vi "debug.vi"() -> ()   [LabVIEW 2010, in "LASA Beta.lvrbt"]
uses:
  LASA Beta.lvrbt
  <vilib>/NXT/Block Support/NXT_ButtonSelector.ctl
  <vilib>/NXT/Dual Mode Library/Display/clearDisplay.vi
  <vilib>/NXT/Dual Mode Library/Display/drawText.vi
  <vilib>/NXT/Dual Mode Library/Sensors/readNXTButton.vi
  op-run.vi
  <vilib>/NXT/Dual Mode Library/prims/inRangeAndCoerce/inRangeAndCoerce_float.vi
panel:
  in  "Manipulator position":dbl=127.0
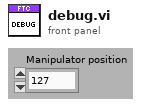
[diagram p1: front panel]
types:
  T1 = typedef "LVHSConnector.ctl" = cluster{"Hardware":string, "Flattened String":string}
  T2 = typedef "NXT_ButtonSelector.ctl" = u16
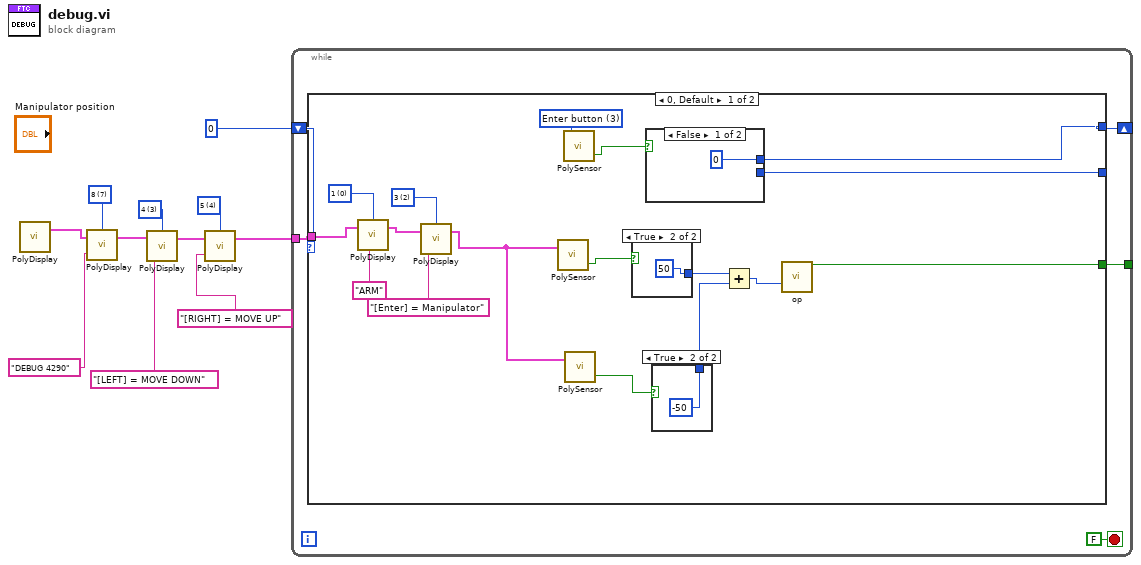
[diagram p0: block diagram]
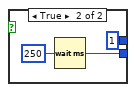
[diagram p4: hidden frame]
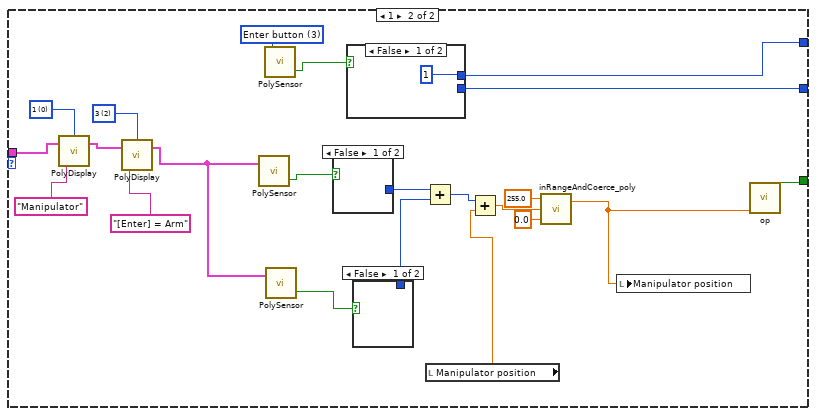
[diagram p5: hidden frame]
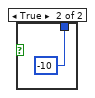
[diagram p6: hidden frame]
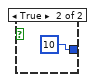
[diagram p7: hidden frame]
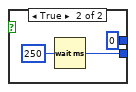
[diagram p8: hidden frame]
diagram:
  w6 = i16 7 items=["1", "2", "3", "4", "5", "6", "7", "8"] ("Line")
  w7 = i16 3 items=["1", "2", "3", "4", "5", "6", "7", "8"] ("Line")
  w8 = i16 4 items=["1", "2", "3", "4", "5", "6", "7", "8"] ("Line")
  n1 = call-poly <vilib>:"PolyDisplay.vi"() -> ("NXT"=w11:T1)  [unwired: 4 in]
  n2 = call-poly <vilib>:"PolyDisplay.vi"("Text"="DEBUG 4290", "NXT"=w11, "Line"=w6) -> ("NXT"=w10:T1)  [unwired: 1 in]
  n3 = call-poly <vilib>:"PolyDisplay.vi"("Text"="[LEFT] = MOVE DOWN", "NXT"=w10, "Line"=w7) -> ("NXT"=w9:T1)  [unwired: 1 in]
  n4 = call-poly <vilib>:"PolyDisplay.vi"("Text"="[RIGHT] = MOVE UP", "NXT"=w9, "Line"=w8) -> ("NXT"=w1:T1)  [unwired: 1 in]
  n5 = while {
    shift-right: [w14] -> _
    shift-left: 0 -> [w15]
    tunnel: w1 -> [w13]
    tunnel: [w12] -> _
    stop <- FALSE stop-if-true
    n6 = case shown="0, Default" w15 {
      tunnel: [w24 w52] -> w14
      tunnel: w13 -> [w33 w61]
      tunnel: [w25 w53] -> _
      tunnel: [w17 w46] -> w12
      frame 0, Default {
        w27 = T2 3 items=["Enter button"=3, "Left button"=2, "Right button"=1] ("Button (Enter button)")
        w30 = i16 2 items=["1", "2", "3", "4", "5", "6", "7", "8"] ("Line")
        w32 = i16 0 items=["1", "2", "3", "4", "5", "6", "7", "8"] ("Line")
        n7 = call-poly <vilib>:"PolyDisplay.vi"("Text"="ARM", "NXT"=w33, "Line"=w32) -> ("NXT"=w28:T1)  [unwired: 1 in]
        n8 = call-poly <vilib>:"PolyDisplay.vi"("Text"="[Enter] = Manipulator", "NXT"=w28, "Line"=w30) -> ("NXT"=w23:T1)  [unwired: 1 in]
        n9 = call-poly <vilib>:"PolySensor.vi"("NXT"=w23) -> ("Yes/No"=w21:bool)  [unwired: 2 in, 1 out]
        n10 = call-poly <vilib>:"PolySensor.vi"("Button (Enter button)"=w27) -> ("Yes/No"=w26:bool)  [unwired: 2 in, 1 out]
        n11 = call-poly <vilib>:"PolySensor.vi"("NXT"=w23) -> ("Yes/No"=w22:bool)  [unwired: 2 in, 1 out]
        n12 = case shown="True" w21 {
          tunnel: [_ 50] -> w20
          frame False {
          }
          frame True {
          }
        }
        n13 = case shown="False" w26 {
          tunnel: [_ w39] -> w25
          tunnel: [0 1] -> w24
          frame False {
          }
          frame True {
            n14 = Wait (ms)(milliseconds to wait=u32 250) -> (millisecond timer value=w39:u32)
          }
        }
        n15 = case shown="True" w22 {
          tunnel: [_ -50] -> w19
          frame False {
          }
          frame True {
          }
        }
        n16 = Add(x=w20, y=w19) -> (x+y=w18:i32)
        n17 = call-poly "op.vi"("Arm"=w18) -> ("Chain OUT"=w17:bool)  [unwired: 14 in]
      }
      frame 1 {
        w55 = T2 3 items=["Enter button"=3, "Left button"=2, "Right button"=1] ("Button (Enter button)")
        w58 = i16 2 items=["1", "2", "3", "4", "5", "6", "7", "8"] ("Line")
        w60 = i16 0 items=["1", "2", "3", "4", "5", "6", "7", "8"] ("Line")
        n18 = call-poly <vilib>:"PolyDisplay.vi"("Text"="Manipulator", "NXT"=w61, "Line"=w60) -> ("NXT"=w56:T1)  [unwired: 1 in]
        n19 = call-poly <vilib>:"PolyDisplay.vi"("Text"="[Enter] = Arm", "NXT"=w56, "Line"=w58) -> ("NXT"=w51:T1)  [unwired: 1 in]
        n20 = call-poly <vilib>:"PolySensor.vi"("NXT"=w51) -> ("Yes/No"=w49:bool)  [unwired: 2 in, 1 out]
        n21 = call-poly <vilib>:"PolySensor.vi"("Button (Enter button)"=w55) -> ("Yes/No"=w54:bool)  [unwired: 2 in, 1 out]
        n22 = call-poly <vilib>:"PolySensor.vi"("NXT"=w51) -> ("Yes/No"=w50:bool)  [unwired: 2 in, 1 out]
        n23 = case shown="False" w49 {
          tunnel: [_ 10] -> w48
          frame False {
          }
          frame True {
          }
        }
        n24 = case shown="False" w54 {
          tunnel: [_ w67] -> w53
          tunnel: [1 0] -> w52
          frame False {
          }
          frame True {
            n25 = Wait (ms)(milliseconds to wait=u32 250) -> (millisecond timer value=w67:u32)
          }
        }
        n26 = case shown="False" w50 {
          tunnel: [_ -10] -> w47
          frame False {
          }
          frame True {
          }
        }
        n27 = Add(x=w48, y=w47) -> (x+y=w45:i32)
        n28 = local read "Manipulator position"() -> (w44:dbl)
        n29 = Add(x=w45, y=w44) -> (x+y=w43:dbl)
        n30 = call-poly <vilib>:"inRangeAndCoerce_poly.vi"("lower limit"=0.0, "x"=w43, "upper limit"=255.0) -> ("coerced(x)"=w40:dbl)  [unwired: 1 out]
        n31 = local write "Manipulator position"(w40) -> ()
        n32 = call-poly "op.vi"("Manipulator Position"=w40) -> ("Chain OUT"=w46:bool)  [unwired: 14 in]
      }
    }
  }
